vi "Initialise settings.vi"(8 "error in (no error)":errorcluster, 11 "ServiceManager in":refnum<class "ServiceManager.lvclass">) -> (0 "error out":errorcluster, 3 "ServiceManager out":refnum<class "ServiceManager.lvclass">)   [LabVIEW 2012, in "ServiceManager.lvclass"]
uses:
  ServiceManager.lvclass
  settings_enum.ctl
  ServiceManager.lvclass/ServiceManager.ctl
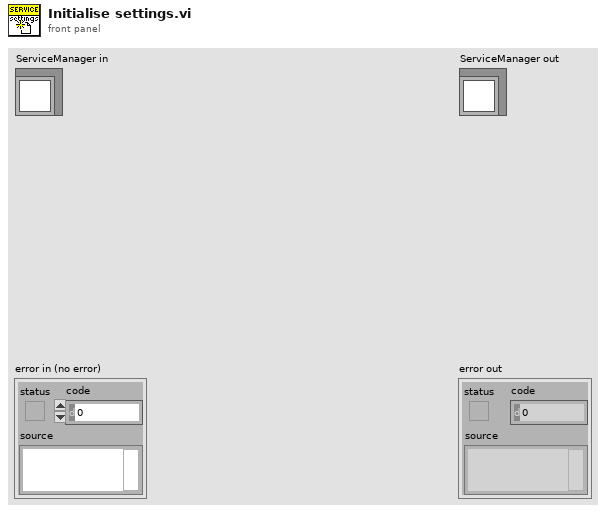
[diagram p1: front panel]
types:
  T1 = typedef "ServiceManager.lvclass/settings_enum.ctl" = string
  T2 = typedef "ServiceManager.lvclass/configuration_enum.ctl" = string
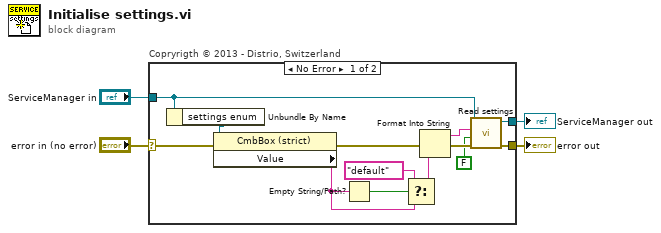
[diagram p0: block diagram]
diagram:
  n1 = case "Copryrigth © 2013 - Distrio, Switzerland" shown="No Error" "error in (no error)" {
    selector: "error in (no error)" -> [w16 w19]
    tunnel: [w7 w19] -> w3
    tunnel: [w6 w18] -> w1
    tunnel: "ServiceManager in" -> [w12 w18]
    frame No Error {
      n2 = Unbundle By Name(w12) -> ("settings enum"=w17:refnum<vi>)
      n3 = property class="CmbBox (strict)"(reference=w17, error in=w16) -> (error out=w9:errorcluster, "Value"=w14:T2)  [unwired: 1 out]
      n4 = Empty String/Path?(string/path=w14) -> (empty?=w15:bool)
      n5 = Select(t=T1 "default", s=w15, f=w14) -> (s? t:f=w10:T2)
      n6 = Format Into String(error in=w9, w10) -> (resulting string=w11:string, error out=w8:errorcluster)  [unwired: 2 in]
      n7 = call-dynamic "Read settings.vi"("error in (no error)"=w8, "force loading?"=FALSE, "settings name"=w11, "ServiceManager in"=w12) -> ("error out"=w7:errorcluster, "ServiceManager out"=w6:refnum<class "ServiceManager.lvclass">)  [unwired: 4 in, 2 out]
    }
    frame Error {
    }
  }
  "error out" <- w3
  "ServiceManager out" <- w1
